vi "svfa_Process Coherence.vi"(0 "Windowed signal [X]":dbl[](array[numeric]) format="%.2f", 1 "processing control":T1(ring), 5 "Windowed signal [Y]":dbl[](array[numeric]) format="%.2f", 7 "dt":dbl format="%.2f", 9 "averaging parameters":T2={"averaging mode"=enum."No averaging", "weighting mode"=enum."Linear", "number of averages"=10, "linear mode"=enum."Auto restart"}, 11 "error in (no error)":errorcluster) -> (2 "averaging done":bool, 3 "averages completed":dbl format="%.2f", 4 "Coherence":dbl[](array[numeric]) format="%.2f", 6 "<Gxx>":dbl[](array[numeric]) format="%.2f", 8 "df":dbl format="%.2f", 10 "<Gyy>":dbl[](array[numeric]) format="%.2f", 13 "MAG <Gxy>":dbl[](array[numeric]) format="%.2f", 14 "PHASE <Gxy>":dbl[](array[numeric]) format="%.2f", 15 "error out":errorcluster)   [LabVIEW 2017]
uses:
  <vilib>/Analysis/2dsp.llb/Power Spectrum (DBL).vi
  <vilib>/Analysis/2dsp.llb/Cross Power (DBL).vi
  <vilib>/addons/_NISVFA/_Shared subVIs/Spectrum Averaging/svfa_Reset Averaging State Info.vi
  <vilib>/addons/_NISVFA/_Shared subVIs/Spectrum Averaging/svfa_Average Array with Avg Checks (complex) No State.vi
  <vilib>/addons/_NISVFA/_Shared subVIs/Spectrum Averaging/svfa_Average Array with Avg Checks (real) No State.vi
  <vilib>/addons/_NISVFA/_Shared subVIs/Spectrum Averaging/svfa_Average Array (complex) No State.vi
  <vilib>/addons/_NISVFA/_Shared subVIs/Spectrum Averaging/svfa_Average Array (real) No State.vi
  <vilib>/addons/_NISVFA/_Shared subVIs/Spectrum Averaging/svfa_No Average Array (complex).vi
  <vilib>/addons/_NISVFA/_Shared subVIs/Spectrum Averaging/svfa_Average Array (complex).vi
  <vilib>/addons/_NISVFA/_Shared subVIs/Spectrum Averaging/svfa_Average Array (real).vi
  <vilib>/addons/_NISVFA/_Shared subVIs/Spectrum Averaging/svfa_Peak Hold Array.vi
  <vilib>/Analysis/NI_AALPro.lvlib
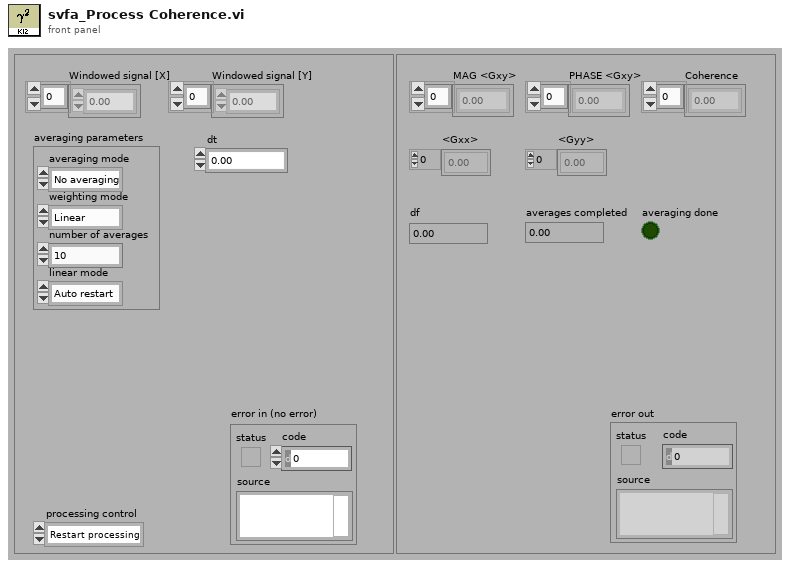
[diagram p1: front panel]
types:
  T1 = enum16{"Restart processing", "Continue processing", "Skip processing"}
  T2 = cluster{"averaging mode":enum16{"No averaging", "Vector averaging", "RMS averaging", "Peak hold"}, "weighting mode":enum16{"Linear", "Exponential"}, "number of averages":u32, "linear mode":enum16{"One shot", "Auto restart"}}
  T3 = enum16{"No averaging", "Vector averaging", "RMS averaging", "Peak hold"}
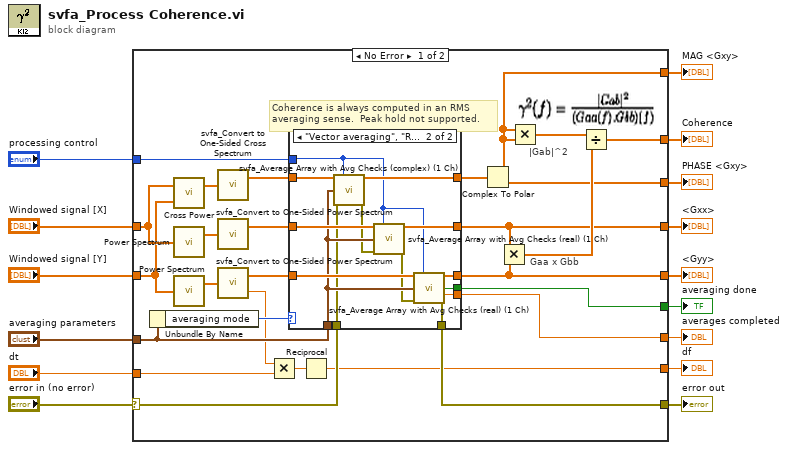
[diagram p0: block diagram]
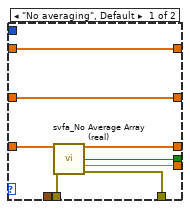
[diagram p2: hidden frame]
diagram:
  n1 = case shown="No Error" "error in (no error)" {
    selector: "error in (no error)" -> [w28 w65]
    tunnel: "Windowed signal [X]" -> [w24 _]
    tunnel: "Windowed signal [Y]" -> [w20 _]
    tunnel: "dt" -> [w18 _]
    tunnel: [w29 _] -> w12
    tunnel: [w38 _] -> w10
    tunnel: [w37 _] -> w9
    tunnel: [w36 _] -> w8
    tunnel: [w35 _] -> w7
    tunnel: [w34 _] -> w6
    tunnel: "averaging parameters" -> [w31 _]
    tunnel: [w17 _] -> w4
    tunnel: "processing control" -> [w33 _]
    tunnel: [w32 w65] -> w1
    tunnel: [w40 _] -> w11
    frame No Error {
      # "Coherence is always computed in an RMS\naveraging sense.  Peak hold not supported."
      # "|Gab|^2"
      # "Gaa x Gbb"
      n2 = Unbundle By Name(w31) -> ("averaging mode"=w30:T3)
      n3 = call-poly <vilib>:"Cross Power.vi"("Y"=w20, "X"=w24) -> ("Sxy"=w25:cdb[])  [unwired: 1 out]
      n4 = call-poly <vilib>:"Power Spectrum.vi"("X"=w24) -> ("Power Spectrum"=w27:dbl[])  [unwired: 1 out]
      n5 = call-poly <vilib>:"Power Spectrum.vi"("X"=w20) -> ("Power Spectrum"=w22:dbl[])  [unwired: 1 out]
      n6 = call <vilib>:"svfa_Convert to One-Sided Cross Spectrum.vi"("two-sided cross spectrum"=w25) -> ("one-sided cross spectrum"=w23:cdb[])  [unwired: 1 out]
      n7 = call <vilib>:"svfa_Convert to One-Sided Power Spectrum.vi"("two-sided power spectrum"=w27) -> ("one-sided power spectrum"=w26:dbl[])  [unwired: 1 out]
      n8 = call <vilib>:"svfa_Convert to One-Sided Power Spectrum.vi"("two-sided power spectrum"=w22) -> ("one-sided power spectrum"=w21:dbl[], "block size"=w19:dbl)
      n9 = Multiply(x=w19, y=w18) -> (x*y=w16:dbl)
      n10 = case shown="\"Vector averaging\", \"RMS averaging\"" w30 {
        tunnel: w23 -> [w50 w64]
        tunnel: w26 -> [w49 w63]
        tunnel: w21 -> [w48 w62]
        tunnel: [w50 w61] -> w39
        tunnel: [w49 w60] -> w38
        tunnel: [w45 w59] -> w37
        tunnel: [w47 w58] -> w36
        tunnel: [w46 w57] -> w34
        tunnel: w31 -> [_ w56]
        tunnel: w33 -> [_ w55]
        tunnel: w28 -> [w44 w54]
        tunnel: [w43 w51] -> w32
        frame "No averaging", Default {
          n11 = call <vilib>:"svfa_No Average Array (real).vi"("spectrum"=w48, "error in (no error)"=w44) -> ("dup spectrum"=w47:dbl[], "averaging done"=w45:bool, "averages completed"=w46:dbl, "error out"=w43:errorcluster)  [unwired: 9 in, 1 out]
        }
        frame "Vector averaging", "RMS averaging" {
          n12 = call <vilib>:"svfa_Average Array with Avg Checks (complex) (1 Ch).vi"("spectrum"=w64, "processing control"=w55, "averaging parameters"=w56, "error in (no error)"=w54) -> ("average spectrum"=w61:cdb[], "error out"=w52:errorcluster)  [unwired: 7 in, 3 out]
          n13 = call <vilib>:"svfa_Average Array with Avg Checks (real) (1 Ch).vi"("spectrum"=w63, "processing control"=w55, "averaging parameters"=w56, "error in (no error)"=w52) -> ("average spectrum"=w60:dbl[], "error out"=w53:errorcluster)  [unwired: 7 in, 3 out]
          n14 = call <vilib>:"svfa_Average Array with Avg Checks (real) (1 Ch).vi"("spectrum"=w62, "processing control"=w55, "averaging parameters"=w56, "error in (no error)"=w53) -> ("average spectrum"=w58:dbl[], "averaging done"=w59:bool, "averages completed"=w57:dbl, "error out"=w51:errorcluster)  [unwired: 7 in, 1 out]
        }
      }
      n15 = Reciprocal(x=w16) -> (1/x=w17:dbl)
      n16 = Complex To Polar(r * e^(i*theta)=w39) -> (r=w29:dbl[], theta=w35:dbl[])
      n17 = Multiply(x=w38, y=w36) -> (x*y=w42:dbl[])
      n18 = Multiply(x=w29, y=w29) -> (x*y=w41:dbl[])
      n19 = Divide(x=w41, y=w42) -> (x/y=w40:dbl[])
    }
    frame Error {
    }
  }
  "Coherence" <- w11
  "averaging done" <- w9
  "<Gxx>" <- w10
  "<Gyy>" <- w8
  "MAG <Gxy>" <- w12
  "PHASE <Gxy>" <- w7
  "averages completed" <- w6
  "df" <- w4
  "error out" <- w1
